vi "Emergency_stop_and_Reset.vi"() -> ()   [LabVIEW 2017]
panel:
  out "E-Stop status":picture
  out "Response time":u32
  out "Test Result status":picture
  out "XY Graph":cluster{dbl, u32}[](graph)
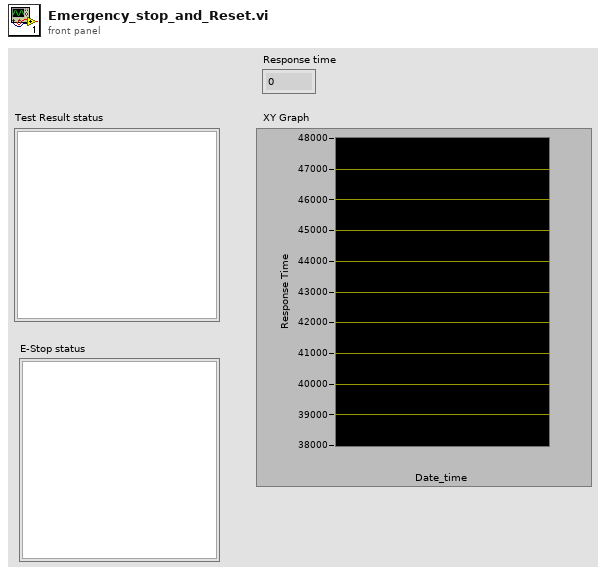
[diagram p1: front panel]
types:
  T1 = enum16{"open", "replace", "create", "open or create", "replace or create", "replace or create with confirmation"}
  T2 = cluster{"[0]":string, "[1]":string, "[2]":string, "[3]":string, "[4]":string, "[5]":string, "[6]":string, "[7]":string, "[8]":string}
  T3 = cluster{"Iterations":u32, "DelayBetweenIterations":u32, "Timeout":u32, "USB6008Port":string, "ActiveLow":i32, "DelayToResetEstop":i32, "ActiveHigh":i32, "Trigger_source":string, "SamplesRate":i32, "Timestamp":string, "TestSuite":string, "ReportPath":path, "FWVersionPath":path}
  T4 = cluster{"Socket_IP_Address":string, "Socket_Port_Number":u16, "Global_ReportPath":path}
  T5 = typedef "imagedata.ctl" = cluster{"image type":i32, "image depth":i32, "image":u8[], "mask":u8[], "colors":u32[], "Rectangle":cluster{"left":i16, "top":i16, "right":i16, "bottom":i16}}
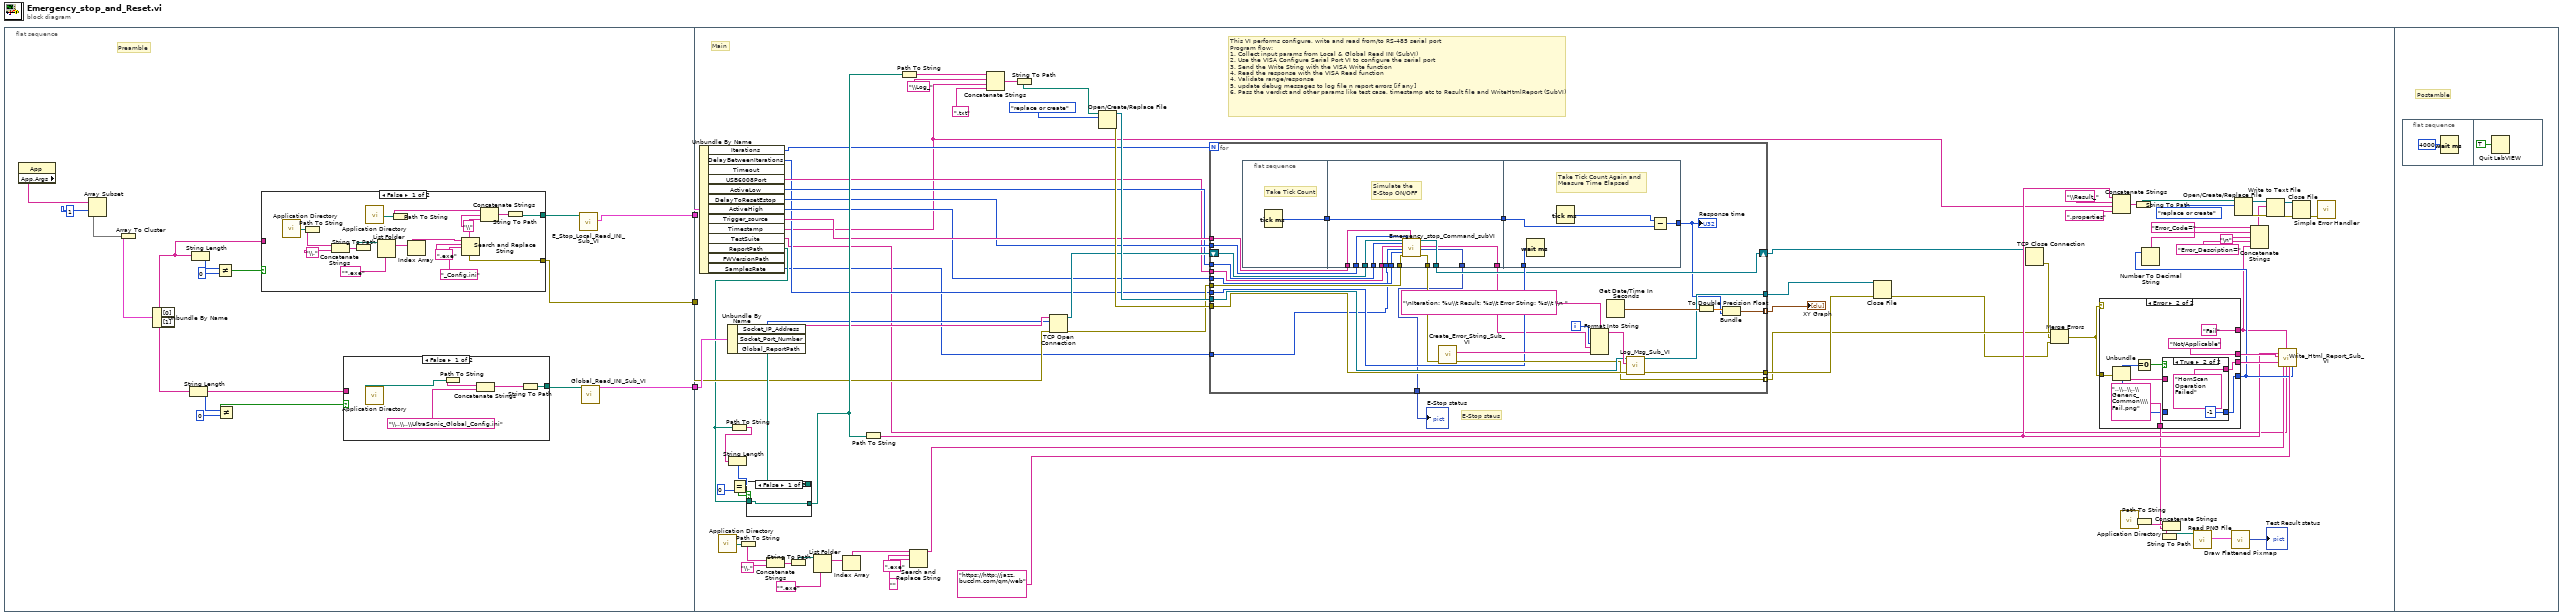
[diagram p0: block diagram]
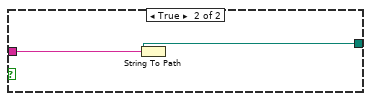
[diagram p2: hidden frame]
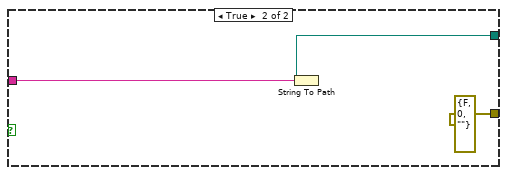
[diagram p3: hidden frame]
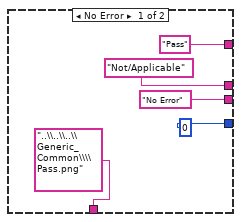
[diagram p5: hidden frame]
diagram:
  n1 = flat-sequence {
    tunnel: [w6] -> w3
    tunnel: [w5] -> w2
    tunnel: [w4] -> w1
    tunnel: w3 -> [w66]
    tunnel: w2 -> [w71]
    tunnel: w1 -> [w61]
    frame #0 {
      # "Preamble"
      n2 = property class="App"() -> ("App.Args"=w8:string[])  [unwired: 2 in, 2 out]
      n3 = Array Subset "Array Subset"(array=w8, index=1) -> (w9:string[])  [unwired: 1 in]
      n4 = Array To Cluster(array=w9) -> (cluster=w10:T2)
      n5 = Unbundle By Name "Unbundle By Name"(w10) -> ("[0]"=w14:string, "[1]"=w17:string)
      n6 = String Length(string=w17) -> (length=w18:i32)
      n7 = String Length(string=w14) -> (length=w11:i32)
      n8 = Not Equal?(x=w11, y=0) -> (x != y?=w13:bool)
      n9 = Not Equal?(x=w18, y=0) -> (x != y?=w16:bool)
      n10 = case shown="False" w13 {
        tunnel: w14 -> [_ w47]
        tunnel: [w29 w46] -> w19
        tunnel: [w28 errorcluster {"status"=FALSE, "code"=0, "source"=""} ("error out")] -> w6
        frame False {
          n11 = call <vilib>:"Application Directory.vi"() -> ("Application Directory"=w35:path)
          n12 = Path To String(path=w35) -> (string=w34:string)
          n13 = Concatenate Strings(w34, "\\." ("string")) -> (w32:string)
          n14 = String To Path(string=w32) -> (path=w37:path)
          n15 = call <vilib>:"Application Directory.vi"() -> ("Application Directory"=w44:path)
          n16 = List Folder(path=w37, pattern="*.exe") -> (filenames=w31:string[])  [unwired: 2 in, 3 out]
          n17 = Path To String(path=w44) -> (string=w39:string)
          n18 = Index Array(array=w31) -> (element=w30:string)  [unwired: 1 in]
          n19 = Search and Replace String(input string=w30, search string=".exe", replace string="_Config.ini" ("replace string (\"\")")) -> (result string=w41:string, error out=w28:errorcluster)  [unwired: 5 in, 2 out]
          n20 = Concatenate Strings(w39, "\\" ("string"), w41) -> (w38:string)
          n21 = String To Path(string=w38) -> (path=w29:path)
        }
        frame True {
          n22 = String To Path(string=w47) -> (path=w46:path)
        }
      }
      n23 = case shown="False" w16 {
        tunnel: [w22 w27] -> w20
        tunnel: w17 -> [_ w26]
        frame False {
          n24 = call <vilib>:"Application Directory.vi"() -> ("Application Directory"=w21:path)
          n25 = Path To String(path=w21) -> (string=w25:string)
          n26 = Concatenate Strings(w25, "\\..\\..\\UltraSonic_Global_Config.ini" ("string")) -> (w23:string)
          n27 = String To Path(string=w23) -> (path=w22:path)
        }
        frame True {
          n28 = String To Path(string=w26) -> (path=w27:path)
        }
      }
      n29 = call "E_Stop_Local_Read_INI_Sub_VI.vi"("Config File Path"=w19) -> ("E-stop Parameters"=w4:T3)  [unwired: 10 in]
      n30 = call "Global_Read_INI_Sub_VI.vi"("Config File Path"=w20) -> ("output cluster"=w5:T4)  [unwired: 14 in]
    }
    frame #1 {
      # "E-Stop staus"
      # "This VI performs configure, write and read from/to RS-485 serial port\nProgram flow:\n1. Collect input params from Local & Global Read INI (SubVI)\n2. Use the VISA Configure Serial Port VI to configure the serial port\n3. Send the Write String with the VISA Write function\n4. Read the response with the VISA Read function\n4. Validate range/response\n5. update debug messages to log file n report errors [if any]\n6. Pass the verdict and other params like test case, timestamp etc to Result file and WriteHtmlReport (SubVI)"
      # "Main"
      n31 = Unbundle By Name(w61) -> ("Iterations"=w55:u32, "DelayBetweenIterations"=w54:u32, "USB6008Port"=w57:string, "ActiveLow"=w58:i32, "DelayToResetEstop"=w59:i32, "ActiveHigh"=w56:i32, "Trigger_source"=w60:string, "Timestamp"=w51:string, "TestSuite"=w52:string, "ReportPath"=w53:path, "SamplesRate"=w50:i32)  [unwired: 2 out]
      n32 = call <vilib>:"Application Directory.vi"() -> ("Application Directory"=w87:path)
      n33 = Unbundle By Name(w71) -> ("Socket_IP_Address"=w68:string, "Socket_Port_Number"=w67:u16, "Global_ReportPath"=w70:path)
      n34 = Path To String(path=w53) -> (string=w118:string)
      n35 = String Length(string=w118) -> (length=w117:i32)
      n36 = Equal?(x=w117, y=0) -> (x = y?=w115:bool)
      n37 = Path To String(path=w87) -> (string=w86:string)
      n38 = case shown="False" w115 {
        tunnel: w70 -> [_ w129]
        tunnel: [w128 w129] -> w114
        tunnel: w53 -> [w128 _]
        frame False {
        }
        frame True {
        }
      }
      n39 = Concatenate Strings(w86, "\\." ("string")) -> (w84:string)
      n40 = String To Path(string=w84) -> (path=w89:path)
      n41 = List Folder(path=w89, pattern="*.exe") -> (filenames=w83:string[])  [unwired: 2 in, 3 out]
      n42 = Index Array(array=w83) -> (element=w79:string)  [unwired: 1 in]
      n43 = Path To String(path=w114) -> (string=w91:string)
      n44 = Path To String(path=w114) -> (string=w120:string)
      n45 = Search and Replace String(input string=w79, search string=".exe", replace string="" ("replace string (\"\")")) -> (result string=w82:string)  [unwired: 5 in, 3 out]
      n46 = Concatenate Strings(w120, "\\Log_" ("string"), w51, ".txt" ("string")) -> (w123:string)
      n47 = String To Path(string=w123) -> (path=w122:path)
      n48 = TCP Open Connection(address=w68, remote port or service name=w67, error in (no error)=w66) -> (connection ID=w62:refnum<k5>, error out=w65:errorcluster)  [unwired: 2 in]
      n49 = Open/Create/Replace File(file path (use dialog)=w122, operation (0:open)=T1."replace or create") -> (refnum out=w92:refnum<file>, error out=w95:errorcluster)  [unwired: 1 in, 4 out]
      n50 = for {
        N: w55 -> [_]
        tunnel: w92 -> [w152]
        tunnel: [w151] -> w94
        tunnel: [w149] -> w93
        tunnel: [w154] -> w124 mode=indexing
        tunnel: w95 -> [w150]
        tunnel: [w147] -> w90 mode=indexing
        tunnel: w65 -> [w136]
        shift-right: [w134] -> w63
        shift-left: w62 -> [w142]
        tunnel: w54 -> [w145]
        tunnel: w60 -> [w141]
        tunnel: w59 -> [w140]
        tunnel: w58 -> [w139]
        tunnel: w57 -> [w138]
        tunnel: w56 -> [w137]
        tunnel: w50 -> [w131]
        tunnel: [w130] -> w48
        i -> [w148]
        n51 = flat-sequence {
          tunnel: [w158] -> w144
          tunnel: w144 -> [w171]
          tunnel: [w171] -> w143
          tunnel: w142 -> [w170]
          tunnel: w141 -> [w169]
          tunnel: w140 -> [w168]
          tunnel: w139 -> [w167]
          tunnel: w138 -> [w166]
          tunnel: w137 -> [w165]
          tunnel: w136 -> [w164]
          tunnel: [w163] -> w135
          tunnel: [w162] -> w134
          tunnel: [w161] -> w133
          tunnel: w131 -> [w160]
          tunnel: [w159] -> w130
          tunnel: w143 -> [w175]
          tunnel: [w173] -> w132
          tunnel: w145 -> [w172]
          frame #0 {
            # "Take Tick Count"
            n52 = Tick Count (ms)() -> (millisecond timer value=w158:u32)
          }
          frame #1 {
            # "Simulate the \nE-Stop ON/OFF"
            n53 = call "Emergency_stop_Command_subVI.vi"("TCP connection ID IN"=w170, "Active Low"=w167, "Port"=w166, "Rate"=w160, "dioHigh"=w165, "ERROR IN"=w164, "Delay to reset e-stop"=w168, "Trigger Source"=w169) -> ("TCP Connection \nID out"=w162:refnum<k5>, "E-Stop output"=w161:string, "Estop Test Result"=w159:picture, "ERROR OUT"=w163:errorcluster)  [unwired: 8 in]
          }
          frame #2 {
            # "Take Tick Count Again and Measure Time Elapsed"
            n54 = Wait (ms)(milliseconds to wait=w172) -> ()  [unwired: 1 out]
            n55 = Tick Count (ms)() -> (millisecond timer value=w174:u32)
            n56 = Subtract(x=w174, y=w175) -> (x-y=w173:u32)
          }
        }
        n57 = call "Create_Error_String_Sub_VI.vi"("error in"=w135) -> ("error out"=w147:errorcluster, "Error String"=w146:string)  [unwired: 9 in]
        n58 = Format Into String(format string="\nIteration: %u\\t Result: %s\\t Error String: %s\\t \\n ", w148, w133, w146) -> (resulting string=w153:string)  [unwired: 2 in, 1 out]
        n59 = Get Date/Time In Seconds() -> (seconds since 1Jan1904=w155:timestamp)
        n60 = call "Log_Msg_Sub_VI.vi"("error in (no error)"=w150, "String"=w153, "Byte Stream File in"=w152) -> ("error out"=w149:errorcluster, "Byte Stream File out"=w151:refnum<file>)  [unwired: 7 in]
        n61 = To Double Precision Float(number=w155) -> (double precision float=w156:dbl)
        n62 = Bundle "Bundle"(w156, w132) -> (w154:cluster{dbl, u32})  [unwired: 1 in]
        "Response time" <- w132
      }
      "XY Graph" <- w124
      "E-Stop status" <- w48
      n63 = Close File(refnum=w94, error in=w93) -> (error out=w49:errorcluster)  [unwired: 1 out]
      n64 = TCP Close Connection(connection ID=w63) -> (error out=w64:errorcluster)  [unwired: 2 in, 1 out]
      n65 = Merge Errors "Merge Errors"(w90, w64, w49) -> (w69:errorcluster)
      n66 = case shown="Error" w69 {
        tunnel: ["Pass" "Fail"] -> w96
        tunnel: w69 -> [_ w187]
        tunnel: [0 ("code") w183] -> w100
        tunnel: ["No Error" ("source") w184] -> w127
        tunnel: ["Not/Applicable" "Not/Applicable"] -> w126
        tunnel: ["..\\..\\..\\Generic_Common\\\\Pass.png" ("string") "..\\..\\..\\Generic_Common\\\\Fail.png" ("string")] -> w72
        frame No Error {
        }
        frame Error {
          n67 = Unbundle(w187) -> ("code"=w185:i32, "source"=w181:string)  [unwired: 1 out]
          n68 = Equal To 0?(x=w185) -> (x = 0?=w182:bool)
          n69 = case shown="True" w182 {
            tunnel: [w191 -1 ("code")] -> w183
            tunnel: [w190 "HornScan Operation Failed" ("source")] -> w184
            tunnel: w185 -> [w191 _]
            tunnel: w181 -> [w190 _]
            frame False {
            }
            frame True {
            }
          }
        }
      }
      n70 = Concatenate Strings(w91, "\\Result_" ("string"), w51, ".properties" ("string")) -> (w112:string)
      n71 = call <vilib>:"Application Directory.vi"() -> ("Application Directory"=w73:path)
      n72 = String To Path(string=w112) -> (path=w104:path)
      n73 = Path To String(path=w73) -> (string=w74:string)
      n74 = Number To Decimal String(number=w100) -> (decimal integer string=w99:string)  [unwired: 1 in]
      n75 = Concatenate Strings(w74, w72) -> (w75:string)
      n76 = String To Path(string=w75) -> (path=w78:path)
      n77 = call <vilib>:"Read PNG File.vi"("path to PNG file"=w78) -> ("image data"=w76:T5)  [unwired: 8 in, 2 out]
      n78 = call <vilib>:"Draw Flattened Pixmap.vi"("image data"=w76) -> ("new picture"=→"Test Result status":picture)  [unwired: 8 in]
      n79 = Open/Create/Replace File(file path (use dialog)=w104, operation (0:open)=T1."replace or create") -> (refnum out=w103:refnum<file>, error out=w108:errorcluster)  [unwired: 4 in, 1 out]
      n80 = Concatenate Strings("Error_Code=" ("string"), w99, "\n", "Error_Description=" ("string"), w96) -> (w102:string)
      n81 = Write to Text File(file (use dialog)=w103, text=w102, error in=w108) -> (refnum out=w107:refnum<file>, error out=w106:errorcluster)  [unwired: 1 in, 1 out]
      n82 = call "Write_Html_Report_Sub_VI.vi"("ReprtPath"=w91, "Remarks"=w126, "Error Description"=w127, "TestCase"=w82, "Verdict"=w96, "TestSuite"=w52, "JazzDashboardLink"="https://http://jazz.bucclm.com/qm/web" ("TestSuite"), "Error Code"=w100) -> ()  [unwired: 12 in]
      n83 = Close File(refnum=w107, error in=w106) -> (error out=w105:errorcluster)  [unwired: 1 out]
      n84 = call <vilib>:"Simple Error Handler.vi"("error in (no error)"=w105) -> ()  [unwired: 4 in, 5 out]
    }
    frame #2 {
      # "Postamble"
      n85 = flat-sequence {
        frame #0 {
          n86 = Wait (ms)(milliseconds to wait=u32 4000) -> ()  [unwired: 1 out]
        }
        frame #1 {
          n87 = Quit LabVIEW(quit? (T)=TRUE) -> ()
        }
      }
    }
  }
